vi "temperatura con pmw.vi"() -> ()   [LabVIEW 2020]
uses:
  <vilib>/MakerHub/LINX/Public/Peripherals/Analog/Analog Read 1 Chan.vi
  <vilib>/MakerHub/LINX/Public/Peripherals/PWM/PWM Set Duty Cycle 1 Chan.vi
  <vilib>/MakerHub/LINX/Public/Peripherals/Analog/Analog Read N Chans.vi
  <vilib>/MakerHub/LINX/Private/Local IO/LinxAnalogRead.vi
  <vilib>/MakerHub/LINX/Public/Utilities/Check Channel.vi
  <vilib>/MakerHub/LINX/Public/Utilities/Open Serial.vi
  <vilib>/MakerHub/LINX/Private/Utilties/Generate Error.vi
  <vilib>/MakerHub/LINX/Public/Peripherals/PWM/PWM Set Duty Cycle N Chans.vi
  <vilib>/MakerHub/LINX/LMH-LINX.lvlib
panel:
  in  "PWM Channel":u8
  in  "Analog Channel":u8
  out "Termometro °C":dbl(slide) scale=0.0..100.0
  out "Variaciones de Temperatura":dbl(graph)
  out "Calor":bool
  out "Normal":bool
  out "Frio":bool
  in  "stop":bool
  out "Grados °C":dbl
  in  "Serial Port":refnum<visa-resource-name>
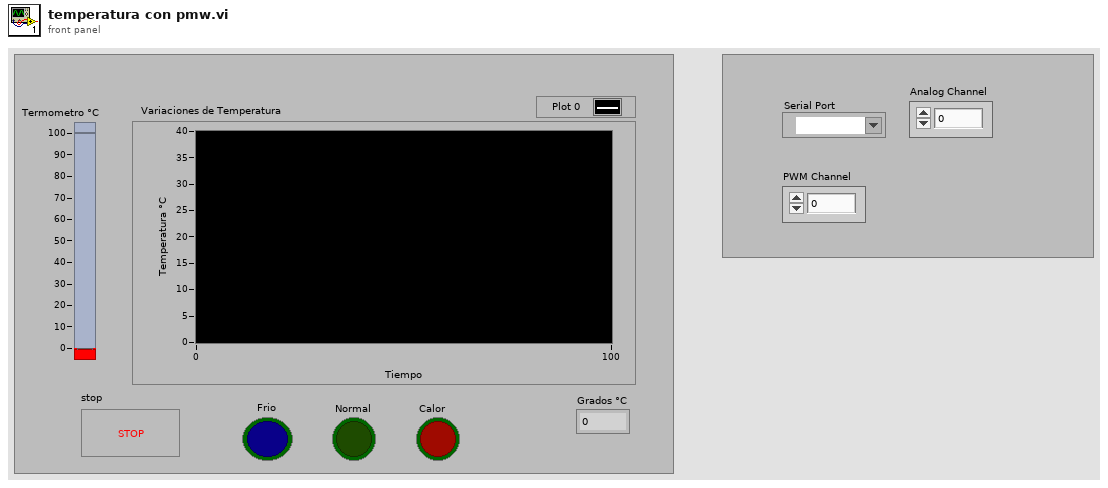
[diagram p1: front panel]
types:
  T1 = typedef "LMH-LINX.lvlib/LINX Ref.ctl" = cluster{"IO":T2, "Interface":T3, "LINX Device Config":T4}
  T2 = typedef "LMH-LINX.lvlib/Platform.ctl" = enum16{"Remote", "Local"}
  T3 = typedef "LMH-LINX.lvlib/Interface.ctl" = enum16{"Serial", "TCP"}
  T4 = typedef "LMH-LINX.lvlib/Device.lvlib/LINX Device Config.ctl" = cluster{"Interface":T3, "COM Port":refnum<visa-resource-name>, "TCP Configuration":T5, "Device Family":u8, "Device ID":u8, "Device Name":string, "TCP Ref":refnum<k5>, "Channels":T6}
  T5 = typedef "LMH-LINX.lvlib/Device.lvlib/TCP Config.ctl" = cluster{"IP Address":string, "Port":u16}
  T6 = typedef "LMH-LINX.lvlib/Channels.ctl" = cluster{"DI":u8[], "DO":u8[], "AI":u8[], "AO":u8[], "PWM":u8[], "QE":u8[], "UART":u8[], "I2C 2":u8[], "SPI":u8[], "CAN":u8[], "Servo":u8[], "AI Ref (V)":dbl, "AI Resolution (Bits)":u8, "AO Ref (V)":dbl, "AO Resolution (Bits)":u8}
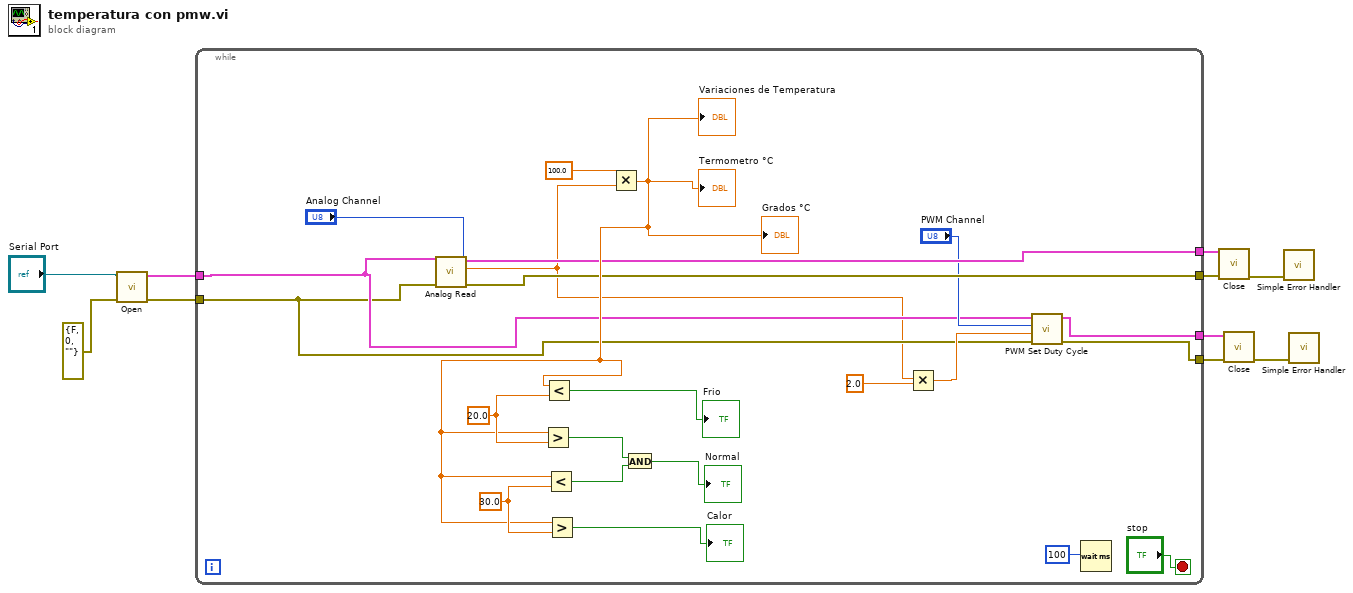
[diagram p0: block diagram]
diagram:
  n1 = call-poly <vilib>:"Open.vi"("Error In"=errorcluster {"status"=FALSE, "code"=0, "source"=""} ("error constant"), "Serial Port"="Serial Port") -> ("Error Out"=w8:errorcluster, "LINX Resource"=w9:T1)  [unwired: 7 in, 1 out]
  n2 = while {
    tunnel: w9 -> [w13]
    tunnel: w8 -> [w12]
    tunnel: [w26] -> w5
    tunnel: [w25] -> w4
    tunnel: [w16] -> w2
    tunnel: [w15] -> w1
    stop <- "stop" stop-if-true
    w31 = 30.0
    w32 = 20.0
    n3 = call-poly <vilib>:"Analog Read.vi"("Error In"=w12, "Analog Channel"="Analog Channel", "LINX Resource"=w13) -> ("Error Out"=w15:errorcluster, "Voltage"=w11:dbl, "LINX Resource"=w16:T1)  [unwired: 5 in, 1 out]
    n4 = Multiply(x=100.0, y=w11) -> (x*y=w20:dbl)
    "Termometro °C" <- w20
    "Variaciones de Temperatura" <- w20
    "Grados °C" <- w20
    n5 = Greater?(x=w20, y=w32) -> (0:w30:bool)
    n6 = Less?(x=w20, y=w32) -> (x < y?=→"Frio":bool)
    n7 = Less?(x=w20, y=w31) -> (x < y?=w29:bool)
    n8 = Greater?(x=w20, y=w31) -> (0:→"Calor":bool)
    n9 = And(x=w30, y=w29) -> (x .and. y?=→"Normal":bool)
    n10 = Multiply(x=w11, y=2.0) -> (x*y=w18:dbl)
    n11 = call-poly <vilib>:"PWM Set Duty Cycle.vi"("Error In"=w12, "Duty Cycle (0-1)"=w18, "PWM Channel"="PWM Channel", "LINX Resource"=w13) -> ("Error Out"=w25:errorcluster, "LINX Resource"=w26:T1)  [unwired: 6 in]
    n12 = Wait (ms)(milliseconds to wait=100) -> ()  [unwired: 1 out]
  }
  n13 = call <vilib>:"Close.vi"("Error In"=w1, "LINX Resource"=w2) -> ("Error Out"=w3:errorcluster)  [unwired: 9 in]
  n14 = call <vilib>:"Close.vi"("Error In"=w4, "LINX Resource"=w5) -> ("Error Out"=w6:errorcluster)  [unwired: 9 in]
  n15 = call <vilib>:"Simple Error Handler.vi"("error in (no error)"=w3) -> ()  [unwired: 4 in, 5 out]
  n16 = call <vilib>:"Simple Error Handler.vi"("error in (no error)"=w6) -> ()  [unwired: 4 in, 5 out]
